vi "CRC校验位1.vi"(1 "输入端":string) -> (0 "CRC校验位":string)   [LabVIEW 2014]
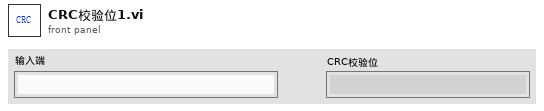
[diagram p1: front panel]
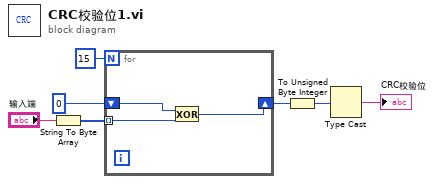
[diagram p0: block diagram]
diagram:
  n1 = String To Byte Array(string="输入端") -> (unsigned byte array=w5:u8[])
  n2 = for {
    N: 15 -> [_]
    tunnel: w5 -> [w10] mode=indexing
    shift-right: [w8] -> w2
    shift-left: u8 0 -> [w9]
    n3 = Exclusive Or(1:w10, 2:w9) -> (0:w8:u8)
  }
  n4 = To Unsigned Byte Integer(number=w2) -> (unsigned 8bit integer=w1:u8)
  n5 = Type Cast(x=w1) -> (*(type *) &x=→"CRC校验位":string)  [unwired: 1 in]
